vi "Update RPM.vi"(8 "error in":errorcluster, 11 "RPMs":dbl[](array[numeric])) -> (0 "error out":errorcluster)   [LabVIEW 2018, in "UDP Writer.lvlib"]
doc: "This subVI enqueues the named action in to the communications queue along with the input data."
uses:
  UDP Writer.lvlib
  Private Controls/Module Data.ctl
  Private Controls/Module Action.ctl
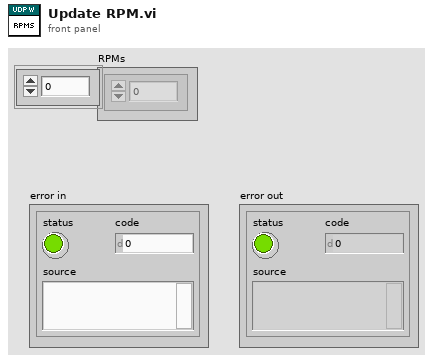
[diagram p1: front panel]
types:
  T1 = typedef "UDP Writer.lvlib/Module Data.ctl" = cluster{"Data":variant, "Action":T2}
  T2 = typedef "UDP Writer.lvlib/Module Action.ctl" = enum16{"Init", "Update ARINC", "Update Waterfall", "Update RPMs", "Update Temps", "Update Modbus", "Update AI", "Update Vibs", "Write", "Error"}
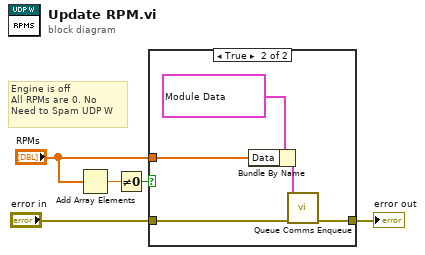
[diagram p0: block diagram]
diagram:
  # "Engine is off\nAll RPMs are 0. No\nNeed to Spam UDP W"
  n1 = Add Array Elements(numeric array="RPMs") -> (sum=w2:dbl)
  n2 = Not Equal To 0?(x=w2) -> (x != 0?=w1:bool)
  n3 = case shown="True" w1 {
    tunnel: [w6 w11] -> w5
    tunnel: "error in" -> [w6 w10]
    tunnel: "RPMs" -> [_ w7]
    frame False {
    }
    frame True {
      n4 = Bundle By Name(cluster=T1 {"Data"=variant, "Action"=enum."Update RPMs"} ("element"), "Data"=w7) -> (w8:T1)
      n5 = call "Queue Comms Enqueue.vi"("error in (no error)"=w10, "element"=w8) -> ("error out"=w11:errorcluster)  [unwired: 9 in]
    }
  }
  "error out" <- w5
